vi "Gear_Ratio_to_Deg_mm.vi"(4 "j4":i32, 5 "j3":i32, 6 "j2":i32, 7 "j1":i32) -> (0 "theta 4":dbl, 1 "theta 3":dbl, 2 "theta 2":dbl, 3 "theta 1":dbl)   [LabVIEW 2016]
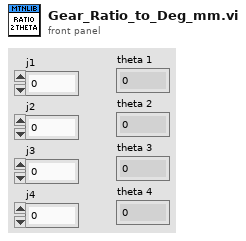
[diagram p1: front panel]
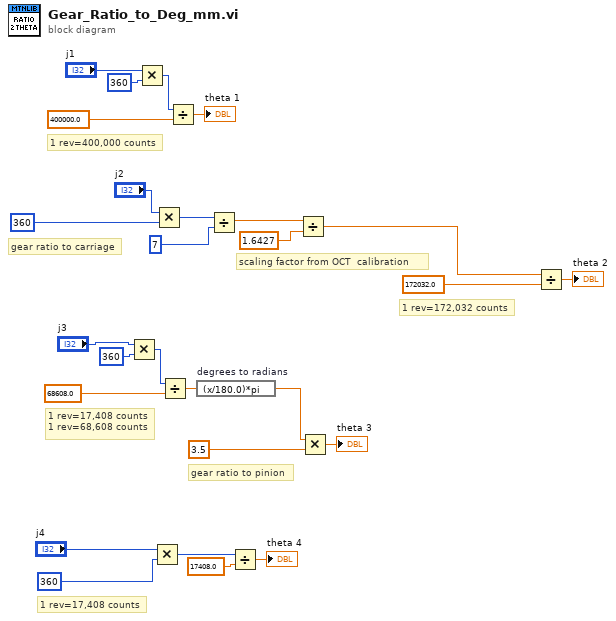
[diagram p0: block diagram]
diagram:
  # "scaling factor from OCT  calibration"
  # "1 rev=17,408 counts"
  # "1 rev=17,408 counts\n1 rev=68,608 counts"
  # "gear ratio to pinion"
  # "gear ratio to carriage"
  # "1 rev=172,032 counts"
  # "1 rev=400,000 counts"
  n1 = Multiply(x="j3", y=360) -> (x*y=w15:i32)
  n2 = Multiply(x="j1", y=360) -> (x*y=w25:i32)
  n3 = Multiply(x="j4", y=360) -> (x*y=w6:i32)
  n4 = Multiply(x="j2", y=360) -> (x*y=w4:i32)
  n5 = Divide(x=w15, y=68608.0) -> (x/y=w13:dbl)
  n6 = Divide(x=w25, y=400000.0) -> (x/y=→"theta 1":dbl)
  n7 = expression code="(x/180.0)*pi" "degrees to radians"(w13) -> (w11:dbl)
  n8 = Divide(x=w4, y=7) -> (x/y=w3:dbl)
  n9 = Divide(x=w6, y=17408.0) -> (x/y=→"theta 4":dbl)
  n10 = Divide(x=w3, y=1.6427) -> (x/y=w19:dbl)
  n11 = Multiply(x=w11, y=3.5) -> (x*y=→"theta 3":dbl)
  n12 = Divide(x=w19, y=172032.0) -> (x/y=→"theta 2":dbl)
